vi "Simultaneous Sound Input Output.vi"() -> ()   [LabVIEW 2017]
doc: "本VI说明如何实现同步声音IO，比如连续播放从麦克风采集的声音数据。需要使用连接至声卡的麦克风。用户可指定输入和输出设备的ID、采样频率以及两个设备的缓冲区大小。频率越高说明质量越好，但将使用更多资源并且受声卡限制。大采样数将有利于减少突波，但会引起采集和播放间的延迟。"
uses:
  <vilib>/sound2/lvsound2.llb/Sampling Mode.ctl
  <vilib>/sound2/lvsound2.llb/Sound Data Format.ctl
  <vilib>/sound2/lvsound2.llb/Sound Output Write (DBL Single).vi
  <vilib>/sound2/lvsound2.llb/Sound Input Read (DBL).vi
  <vilib>/sound2/lvsound2.llb/Sound Output Write (DBL).vi
panel:
  out "采集的声音":waveform(dbl)[](graph)
  in  "停止":bool
  in  "输入设备ID":u32
  in  "输出设备ID":u32
  # "概述：演示使用声音函数连续播放从麦克风采集到的声音。\n要求：麦克风\n操作步骤：\n1. 指定输入设备ID和输出设备ID的值。\n2. 运行VI。\n3.单击停止按钮停止VI。"
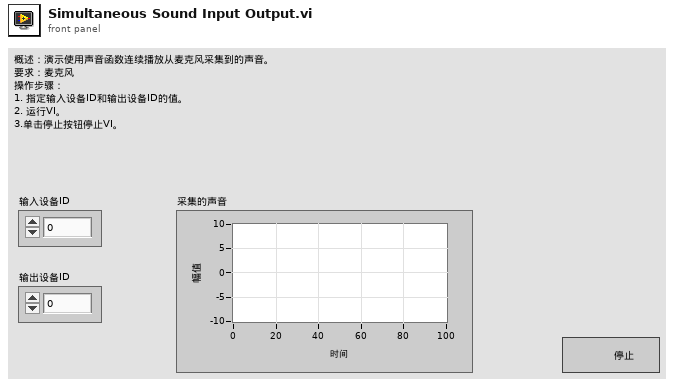
[diagram p1: front panel]
types:
  T1 = typedef "Sound Data Format.ctl" = cluster{"sample rate (S/s)":dbl, "number of channels":i32, "bits per sample":i32}
  T2 = typedef "Sampling Mode.ctl" = i32
  T3 = typedef "Sound Output Task ID.ctl" = u32
  T4 = typedef "Sound Input Task ID.ctl" = u32
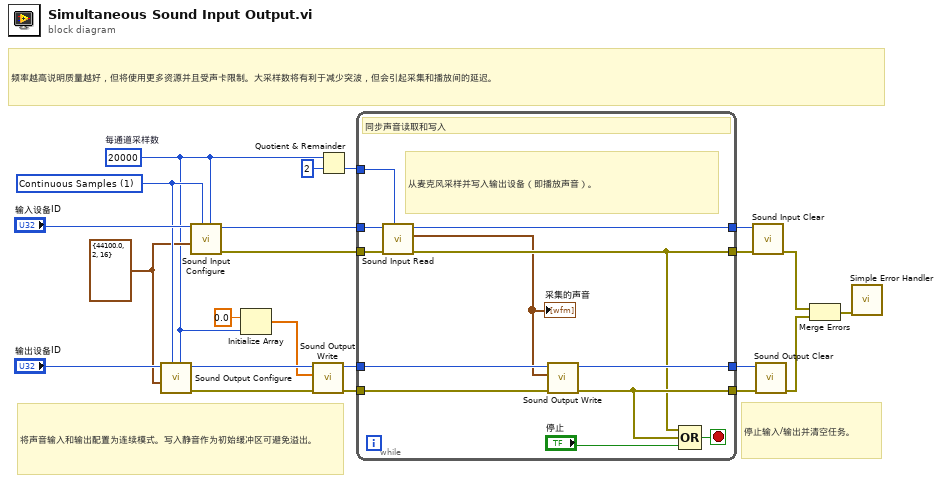
[diagram p0: block diagram]
diagram:
  w2 = 20000  # 每通道采样数
  w6 = T1 {"sample rate (S/s)"=44100.0, "number of channels"=2, "bits per sample"=16} ("Sound Format")
  w12 = T2 1 items=["Finite Samples", "Continuous Samples"] ("sample mode")
  # "频率越高说明质量越好，但将使用更多资源并且受声卡限制。大采样数将有利于减少突波，但会引起采集和播放间的延迟。"
  # "停止输入/输出并清空任务。"
  # "将声音输入和输出配置为连续模式。写入静音作为初始缓冲区可避免溢出。"
  n1 = call <vilib>:"Sound Output Configure.vi"("number of samples/ch"=w2, "sample mode"=w12, "sound format"=w6, "device ID"="输出设备ID") -> ("error out"=w10:errorcluster, "task ID"=w11:T3)  [unwired: 6 in]
  n2 = call <vilib>:"Sound Input Configure.vi"("number of samples/ch"=w2, "sample mode"=w12, "sound format"=w6, "device ID"="输入设备ID") -> ("error out"=w14:errorcluster, "task ID"=w13:T4)  [unwired: 6 in]
  n3 = Initialize Array(0.0 ("element"), w2) -> (w4:dbl[])
  n4 = call-poly <vilib>:"Sound Output Write.vi"("error in (no error)"=w10, "data"=w4, "task ID"=w11) -> ("error out"=w9:errorcluster, "task ID out"=w8:T3)  [unwired: 7 in]
  n5 = Quotient & Remainder(x=w2, y=2) -> (floor(x/y)=w3:i32)  [unwired: 1 out]
  n6 = while {
    tunnel: w3 -> [w30]
    tunnel: w13 -> [w32]
    tunnel: [w29] -> w17
    tunnel: w8 -> [w33]
    tunnel: [w31] -> w20
    tunnel: w9 -> [w28]
    tunnel: [w25] -> w21
    tunnel: w14 -> [w34]
    tunnel: [w24] -> w22
    stop <- w26 stop-if-true
    # "从麦克风采样并写入输出设备（即播放声音）。"
    # "同步声音读取和写入"
    n7 = call-poly <vilib>:"Sound Input Read.vi"("number of samples/ch"=w30, "error in (no error)"=w34, "task ID"=w32) -> ("error out"=w24:errorcluster, "data"=w23:waveform(dbl)[], "task ID out"=w29:T4)  [unwired: 6 in]
    "采集的声音" <- w23
    n8 = call-poly <vilib>:"Sound Output Write.vi"("error in (no error)"=w28, "data"=w23, "task ID"=w33) -> ("error out"=w25:errorcluster, "task ID out"=w31:T3)  [unwired: 7 in]
    n9 = Compound Arithmetic op=OR(w24, w25, "停止") -> (w26:bool)
  }
  n10 = call <vilib>:"Sound Input Clear.vi"("error in (no error)"=w22, "task ID"=w17) -> ("error out"=w15:errorcluster)  [unwired: 9 in]
  n11 = call <vilib>:"Sound Output Clear.vi"("error in (no error)"=w21, "task ID"=w20) -> ("error out"=w16:errorcluster)  [unwired: 9 in]
  n12 = Merge Errors(w15, w16) -> (w7:errorcluster)
  n13 = call <vilib>:"Simple Error Handler.vi"("error in (no error)"=w7) -> ()  [unwired: 4 in, 5 out]
